vi "Assert Trigger.vi"(6 "Trigger # (1)":u32=1 min=1 max=14, 7 "Trigger Type (Digital I/O)":T1(ring), 8 "error in":errorcluster, 10 "Node In":string, 11 "VISA resource name":refnum<visa-resource-name>) -> (0 "error out":errorcluster, 2 "Node Out":string, 3 "VISA resource name out":refnum<visa-resource-name>, 4 "Command String":string)   [LabVIEW 2012, in "Keithley 2600 Series.lvlib"]
doc: "This VI asserts a trigger.\n\n<b>Functions and Attributes Used</b>\ndigio.trigger[n].assert()\ntsplink.trigger[n].assert()\nlan.trigger[n].assert()\ntrigger.set()"
uses:
  Keithley 2600 Series.lvlib
  Private/GlobalVariables.vi
panel:
  # "(c) 2008 Keithley Instruments, Inc.  ALL RIGHTS RESERVED."
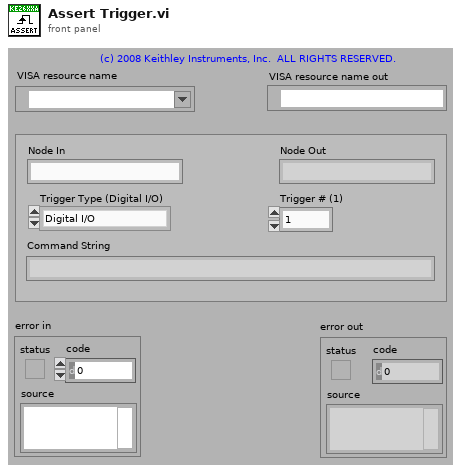
[diagram p1: front panel]
types:
  T1 = enum32{"Digital I/O", "TSP-Link", "LAN", "Software"}
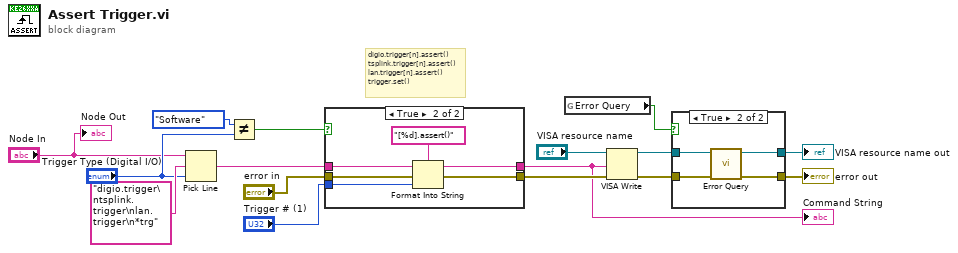
[diagram p0: block diagram]
diagram:
  # "digio.trigger[n].assert()\ntsplink.trigger[n].assert()\nlan.trigger[n].assert()\ntrigger.set()"
  n1 = Pick Line(string ("")="Node In", multi-line string="digio.trigger\ntsplink.trigger\nlan.trigger\n*trg", line index="Trigger Type (Digital I/O)") -> (output string=w13:string)
  n2 = Not Equal?(x=T1."Software", y="Trigger Type (Digital I/O)") -> (x != y?=w9:bool)
  n3 = case shown="True" w9 {
    tunnel: w13 -> [w18 w23]
    tunnel: "Trigger # (1)" -> [_ w22]
    tunnel: "error in" -> [w17 w21]
    tunnel: [w17 w20] -> w8
    tunnel: [w18 w19] -> w1
    frame False {
    }
    frame True {
      n4 = Format Into String(format string="[%d].assert()", initial string=w23, error in=w21, w22) -> (resulting string=w19:string, error out=w20:errorcluster)
    }
  }
  "Command String" <- w1
  n5 = global read "GlobalVariables.vi" "Error Query"() -> (w6:bool)
  n6 = VISA Write(VISA resource name="VISA resource name", write buffer=w1, error in (no error)=w8) -> (VISA resource name out=w5:refnum<visa-resource-name>, error out=w4:errorcluster)  [unwired: 1 out]
  n7 = case shown="True" w6 {
    tunnel: w5 -> [w26 w30]
    tunnel: w4 -> [w25 w29]
    tunnel: [w26 w28] -> w3
    tunnel: [w25 w27] -> w2
    frame False {
    }
    frame True {
      n8 = call "Error Query.vi"("error in (no error)"=w29, "VISA resource name"=w30) -> ("error out"=w27:errorcluster, "VISA resource name out"=w28:refnum<visa-resource-name>)  [unwired: 8 out]
    }
  }
  "VISA resource name out" <- w3
  "error out" <- w2
  "Node Out" <- "Node In"
